vi "FGV_PDU.vi"(8 "errin":errorcluster caption="entrée d'erreur (pas d'erreur)", 9 "Énum":T1, 11 "IN":bool) -> (0 "errout":errorcluster caption="sortie d'erreur", 3 "OUT":bool)   [LabVIEW 2020]
uses:
  ZEN8 Semi Auto EMC/OP700/SubVI/FGV/FGV_Enum.ctl
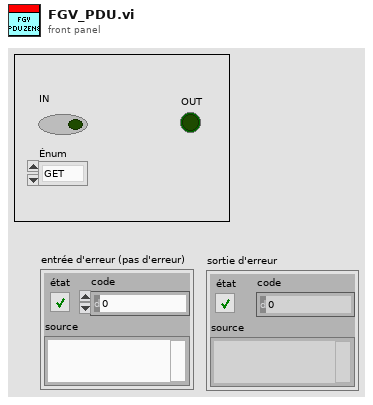
[diagram p1: front panel]
types:
  T1 = typedef "FGV_Enum.ctl" = enum16{"GET", "SET"}
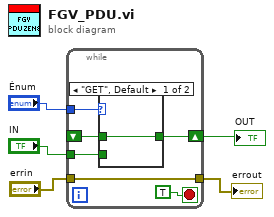
[diagram p0: block diagram]
diagram:
  n1 = while {
    tunnel: "Énum" -> [w10]
    shift-right: [w9] -> w4
    shift-left: _ -> [w8]
    tunnel: "IN" -> [w7]
    tunnel: "errin" -> [w6]
    tunnel: [w6] -> w1
    stop <- TRUE stop-if-true
    n2 = case shown="\"GET\", Default" w10 {
      tunnel: [w12 w13] -> w9
      tunnel: w8 -> [w12 _]
      tunnel: w7 -> [_ w13]
      frame "GET", Default {
      }
      frame "SET" {
      }
    }
  }
  "OUT" <- w4
  "errout" <- w1
